vi "Do.vi"(8 "error in (no error)":errorcluster, 10 "Actor in":refnum<class "Actor.lvclass">, 11 "Show Actor Msg":refnum<class "Show Actor Msg.lvclass">) -> (0 "error out":errorcluster, 2 "Actor out":refnum<class "Actor.lvclass">)   [LabVIEW 2020, in "Msg.lvlib" / "Show Actor Msg.lvclass"]
doc: "This Do implementation will display the front panel of the active actor core clone VI."
uses:
  Show Actor Msg.lvclass
  PPL/HDH.Actor Framework.Core.Actor.lvlibp/1abvi3w/vi.lib/ActorFramework/Actor/Actor.lvclass
  Msg.lvlib
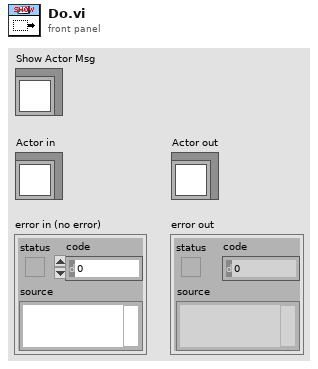
[diagram p1: front panel]
types:
  T1 = enum32{"Invalid", "Standard", "Closed", "Hidden", "Minimized", "Maximized"}
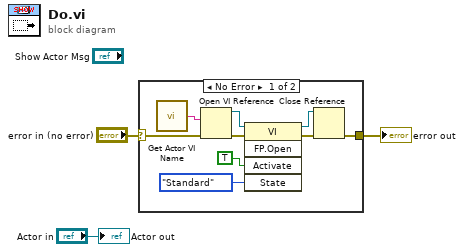
[diagram p0: block diagram]
diagram:
  n1 = case shown="No Error" "error in (no error)" {
    selector: "error in (no error)" -> [w11 w13]
    tunnel: [w4 w13] -> w3
    frame No Error {
      n2 = call "Get Actor VI Name.vi"() -> ("Actor VI Name"=w12:string)
      n3 = Open VI Reference(vi path=w12, error in (no error)=w11) -> (vi reference=w10:refnum<vi>, error out=w7:errorcluster)  [unwired: 4 in]
      n4 = invoke class="VI" method="FP.Open"(reference=w10, error in=w7, "Activate"=TRUE ("Activate?"), "State"=T1."Standard") -> (reference out=w5:refnum<vi>, error out=w6:errorcluster)  [unwired: 1 in, 3 out]
      n5 = Close Reference(reference=w5, error in (no error)=w6) -> (error out=w4:errorcluster)
    }
    frame Error {
    }
  }
  "error out" <- w3
  "Actor out" <- "Actor in"
